vi "End by Reference.vi"(8 "Error In":errorcluster, 11 "Writer In":refnum<data-value>) -> (0 "Error Out":errorcluster, 2 "Data":u8[](array[numeric]), 3 "Writer Out":refnum<data-value>)   [LabVIEW 2019, in "LabPack.lvlib" / "Writer.lvclass"]
uses:
  Writer.lvclass
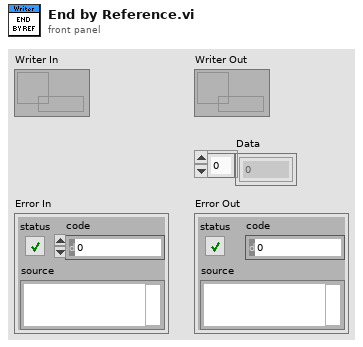
[diagram p1: front panel]
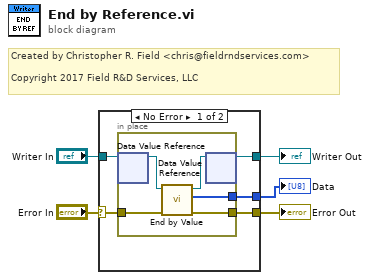
[diagram p0: block diagram]
diagram:
  # "Created by Christopher R. Field <chris@fieldrndservices.com>\n\nCopyright 2017 Field R&D Services, LLC"
  n1 = case shown="No Error" "Error In" {
    selector: "Error In" -> [w8 w17]
    tunnel: [w7 w17] -> w4
    tunnel: "Writer In" -> [w10 w16]
    tunnel: [w9 w16] -> w2
    tunnel: [w6 _] -> w1
    frame No Error {
      n2 = in-place {
        in-place-border: w8 -> [w13]
        in-place-border: [w12] -> w7
        in-place-border: [w11] -> w6
        n3 = in-place-dvr #1(w10) -> (w15:refnum<class "Writer.lvclass">)  [unwired: 1 out]
        n4 = call "End by Value.vi"("Error In"=w13, "Writer In"=w15) -> ("Error Out"=w12:errorcluster, "Data"=w11:u8[], "Writer Out"=w14:refnum<class "Writer.lvclass">)  [unwired: 7 in]
        n5 = in-place-dvr #1(w14) -> (w9:refnum<data-value>)  [unwired: 1 out]
      }
    }
    frame Error {
    }
  }
  "Error Out" <- w4
  "Writer Out" <- w2
  "Data" <- w1
